vi "Msg.vi"(7 "jettl in":refnum<class "jettl.lvclass">, 11 "Last Ack Created Queue Msg Strategy in":refnum<class "Last Ack Created Queue Msg Strategy.lvclass">) -> (5 "jettl out":refnum<class "jettl.lvclass">)   [LabVIEW 2021, in "jettl.lvlib" / "jettl Msg Last Ack Created Queue.lvlib" / "Last Ack Created Queue Msg Strategy.lvclass"]
uses:
  Last Ack Created Queue Msg Strategy.lvclass
  jettl/jettl.lvclass
  jettl Msg Last Ack Created Queue/jettl Msg Last Ack Created Queue.lvclass
  Last Ack Created Queue Msg Strategy.lvclass/Last Ack Created Queue Msg Strategy.ctl
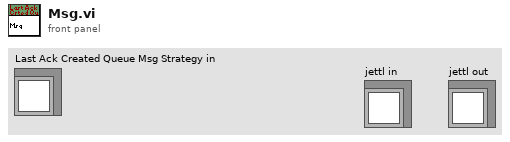
[diagram p1: front panel]
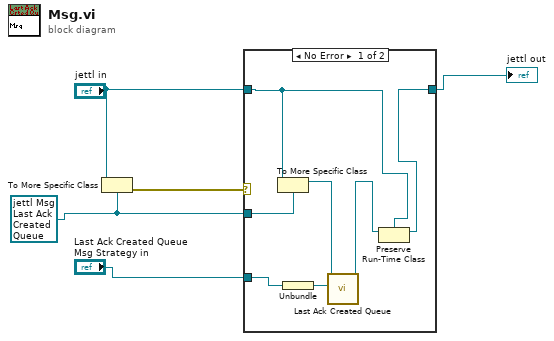
[diagram p0: block diagram]
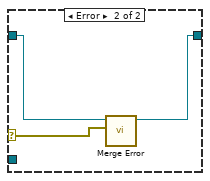
[diagram p2: hidden frame]
diagram:
  w3 = refnum<class "jettl Msg Last Ack Created Queue.lvclass"> refnum ("Last Ack.lvlib:Last Ack.lvclass")
  n1 = To More Specific Class(target class=w3, reference="jettl in") -> (error out=w5:errorcluster)  [unwired: 1 in, 1 out]
  n2 = case shown="No Error" w5 {
    selector: w5 -> [_ w15]
    tunnel: [w6 w13] -> w1
    tunnel: "jettl in" -> [w8 w14]
    tunnel: w3 -> [w12 _]
    tunnel: "Last Ack Created Queue Msg Strategy in" -> [w10 _]
    frame No Error {
      n3 = To More Specific Class(target class=w12, reference=w8) -> (specific class reference=w11:refnum<class "jettl Msg Last Ack Created Queue.lvclass">)  [unwired: 1 in, 1 out]
      n4 = Unbundle(w10) -> (w9:refnum<class "Queue.lvclass">)
      n5 = call-dynamic "Last Ack Created Queue.vi"("Queue"=w9, "jettl Msg Last Ack Created Queue in"=w11) -> ("jettl Msg Last Ack Created Queue out"=w7:refnum<class "jettl Msg Last Ack Created Queue.lvclass">)  [unwired: 9 in]
      n6 = Preserve Run-Time Class(object in=w7, 2:w8) -> (object out=w6:refnum<class "jettl.lvclass">)  [unwired: 1 in, 1 out]
    }
    frame Error {
      n7 = call-dynamic "Merge Error.vi"("Error"=w15, "jettl Msg Merge Error in"=w14) -> ("jettl Msg Merge Error out"=w13:refnum<class "jettl.lvclass">)  [unwired: 9 in]
    }
  }
  "jettl out" <- w1
